vi "Galvo Movimiento Completo.vi"() -> ()   [LabVIEW 2013]
uses:
  <vilib>/DAQmx/write.llb/DAQmx Write (Analog DBL 1Chan 1Samp).vi
  <vilib>/DAQmx/miscellaneous.llb/DAQmx Fill In Error Info.vi
panel:
  in  "Cancel":bool
  in  "start":bool
  in  "milliseconds to wait":u32=10 min=5
  out "error out":errorcluster
  in  "error in":errorcluster
  in  "Stop Button":bool
  in  "Step Angle":sgl=0.1 min=0.01 max=9 step=0.01
  in  "Stop Angle":sgl=2.0 min=-18 max=20 step=0.01
  in  "Start Angle":sgl=-2.0 min=-5 max=5 step=0.01
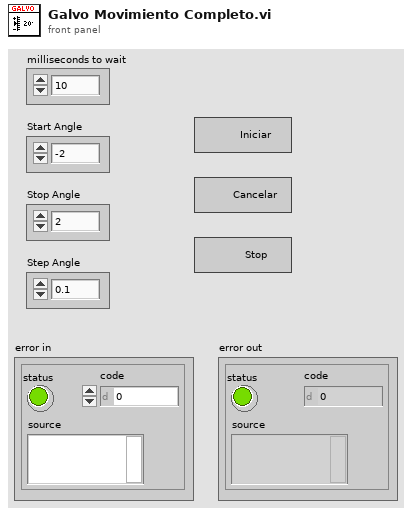
[diagram p1: front panel]
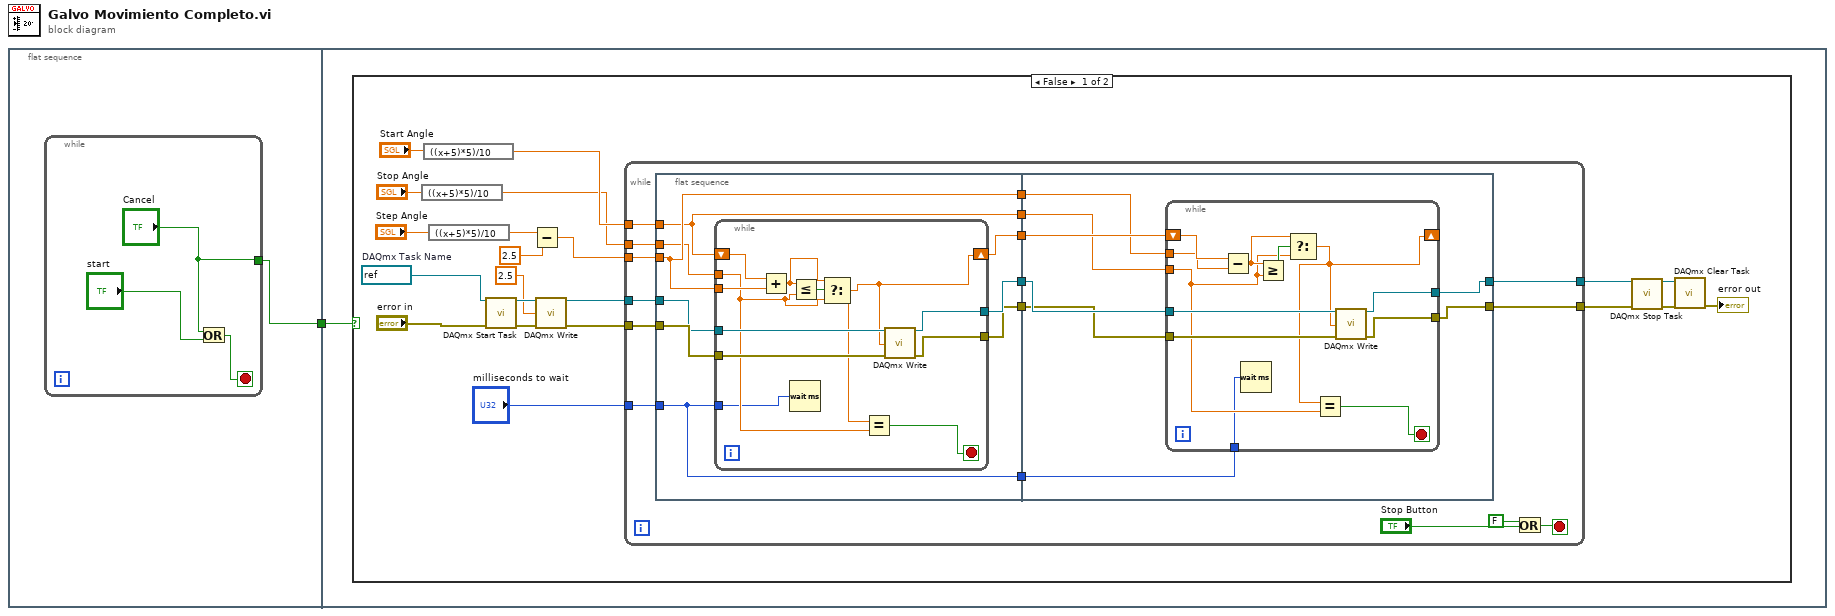
[diagram p0: block diagram]
diagram:
  n1 = flat-sequence {
    tunnel: [w2] -> w1
    tunnel: w1 -> [w6]
    frame #0 {
      n2 = while {
        tunnel: ["Cancel"] -> w2
        stop <- w5 stop-if-true
        n3 = Or(x="Cancel", y="start") -> (x .or. y?=w5:bool)
      }
    }
    frame #1 {
      n4 = case shown="False" w6 {
        frame False {
          w27 = refnum<k21> "EjeX"  # DAQmx Task Name
          n5 = expression code="((x+5)*5)/10"("Stop Angle") -> (w16:sgl)
          n6 = expression code="((x+5)*5)/10"("Start Angle") -> (w18:sgl)
          n7 = expression code="((x+5)*5)/10"("Step Angle") -> (w10:sgl)
          n8 = call <vilib>:"DAQmx Start Task.vi"("task/channels in"=w27, "error in"="error in") -> ("task out"=w25:refnum<k21>, "error out"=w24:errorcluster)  [unwired: 12 in]
          n9 = Subtract(x=w10, y=sgl 2.5) -> (x-y=w8:sgl)
          n10 = call-poly <vilib>:"DAQmx Write.vi"("task/channels in"=w25, "data"=2.5, "error in"=w24) -> ("task out"=w17:refnum<k21>, "error out"=w20:errorcluster)  [unwired: 10 in, 1 out]
          n11 = while {
            tunnel: w20 -> [w41]
            tunnel: w18 -> [w40]
            tunnel: w8 -> [w39]
            tunnel: w17 -> [w38]
            tunnel: w16 -> [w37]
            tunnel: [w36] -> w12
            tunnel: [w35] -> w11
            tunnel: "milliseconds to wait" -> [w29]
            stop <- w44 stop-if-true
            n12 = flat-sequence {
              tunnel: w41 -> [w53]
              tunnel: w40 -> [w46]
              tunnel: w39 -> [w48]
              tunnel: w38 -> [w52]
              tunnel: w37 -> [w47]
              tunnel: [w51] -> w34
              tunnel: [w50] -> w33
              tunnel: [w49] -> w32
              tunnel: [w48] -> w31
              tunnel: [w46] -> w30
              tunnel: w29 -> [w45]
              tunnel: [w45] -> w28
              tunnel: [w72] -> w35
              tunnel: [w73] -> w36
              tunnel: w34 -> [w71]
              tunnel: w33 -> [w70]
              tunnel: w32 -> [w69]
              tunnel: w31 -> [w68]
              tunnel: w30 -> [w67]
              tunnel: w28 -> [w66]
              frame #0 {
                n13 = while {
                  tunnel: w53 -> [w65]
                  tunnel: w48 -> [w63]
                  tunnel: w52 -> [w62]
                  shift-right: [w55] -> w49
                  shift-left: w46 -> [w64]
                  tunnel: w47 -> [w56]
                  tunnel: [w60] -> w51
                  tunnel: [w59] -> w50
                  tunnel: w45 -> [w54]
                  stop <- w61 stop-if-true
                  n14 = Add(x=w64, y=w63) -> (x+y=w57:sgl)
                  n15 = Wait (ms)(milliseconds to wait=w54) -> ()  [unwired: 1 out]
                  n16 = Less Or Equal?(x=w57, y=w56) -> (x <= y?=w58:bool)
                  n17 = Select(t=w57, s=w58, f=w56) -> (s? t:f=w55:sgl)
                  n18 = Equal?(x=w55, y=w56) -> (x = y?=w61:bool)
                  n19 = call-poly <vilib>:"DAQmx Write.vi"("task/channels in"=w62, "data"=w55, "error in"=w65) -> ("task out"=w60:refnum<k21>, "error out"=w59:errorcluster)  [unwired: 10 in, 1 out]
                }
              }
              frame #1 {
                n20 = while {
                  tunnel: w70 -> [w85]
                  tunnel: w67 -> [w76]
                  tunnel: w71 -> [w83]
                  shift-right: [w75] -> _
                  shift-left: w69 -> [w84]
                  tunnel: [w81] -> w73
                  tunnel: [w80] -> w72
                  tunnel: w68 -> [w79]
                  tunnel: w66 -> [w74]
                  stop <- w82 stop-if-true
                  n21 = Subtract(x=w84, y=w79) -> (x-y=w77:sgl)
                  n22 = Wait (ms)(milliseconds to wait=w74) -> ()  [unwired: 1 out]
                  n23 = Greater Or Equal?(x=w77, y=w76) -> (x >= y?=w78:bool)
                  n24 = Select(t=w77, s=w78, f=w76) -> (s? t:f=w75:sgl)
                  n25 = Equal?(x=w75, y=w76) -> (x = y?=w82:bool)
                  n26 = call-poly <vilib>:"DAQmx Write.vi"("task/channels in"=w83, "data"=w75, "error in"=w85) -> ("task out"=w81:refnum<k21>, "error out"=w80:errorcluster)  [unwired: 10 in, 1 out]
                }
              }
            }
            n27 = Or(x=FALSE, y="Stop Button") -> (x .or. y?=w44:bool)
          }
          n28 = call <vilib>:"DAQmx Stop Task.vi"("task/channels in"=w12, "error in"=w11) -> ("task out"=w15:refnum<k21>, "error out"=w14:errorcluster)  [unwired: 12 in]
          n29 = call <vilib>:"DAQmx Clear Task.vi"("task in"=w15, "error in"=w14) -> ("error out"=→"error out":errorcluster)  [unwired: 13 in]
        }
        frame True {
        }
      }
    }
  }
